vi "Register Task.vi"(8 "error in (no error)":errorcluster, 9 "Task ID":string, 10 "EnQr":refnum<class "Message Enqueuer.lvclass">, 11 "VolatusCore in":refnum<class "VolatusCore.lvclass">) -> (0 "error out":errorcluster, 3 "VolatusCore out":refnum<class "VolatusCore.lvclass">)   [LabVIEW 2020, in "Volatus.lvlib" / "VolatusCore.lvclass"]
uses:
  VolatusCore.lvclass
  VolatusCore.lvclass/VolatusCore.ctl
  <vilib>/Utility/miscctls.llb/LVMapReplaceAction.ctl
  <vilib>/ActorFramework/Message Enqueuer/Message Enqueuer.lvclass
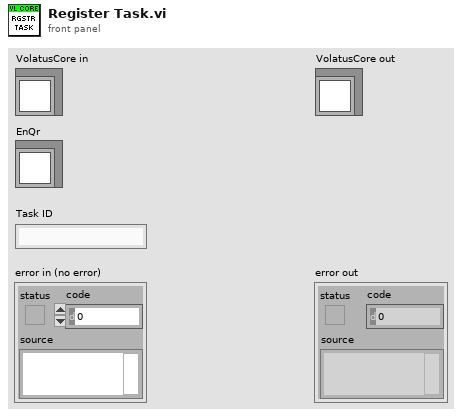
[diagram p1: front panel]
types:
  T1 = typedef "LVMapReplaceAction.ctl" = enum32{"Modify Entry only if found", "Add or Modify Entry", "Delete Entry"}
  T2 = map{string, refnum<class "Message Enqueuer.lvclass">}
  T3 = map{refnum<class "Message Enqueuer.lvclass">, string}
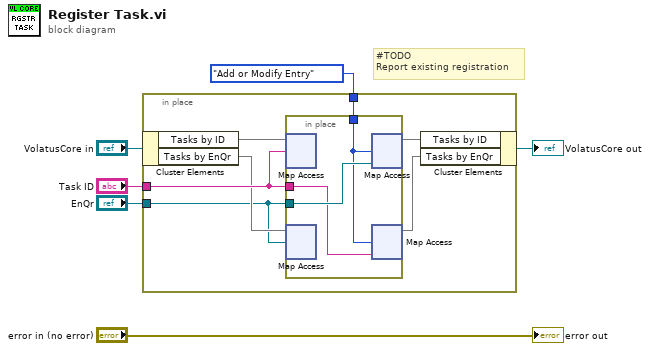
[diagram p0: block diagram]
diagram:
  # "#TODO\nReport existing registration"
  n1 = in-place {
    in-place-border: "Task ID" -> [w12]
    in-place-border: "EnQr" -> [w10]
    in-place-border: LVMapReplaceAction."Add or Modify Entry" ("action") -> [w9]
    n2 = in-place-cluster #1("VolatusCore in") -> ("Tasks by ID"=w13:T2, "Tasks by EnQr"=w11:T3)
    n3 = in-place {
      in-place-border: w12 -> [w15]
      in-place-border: w10 -> [w16]
      in-place-border: w9 -> [w14]
      n4 = in-place-map #2(w13, w12) -> ()  [unwired: 1 in, 2 out]
      n5 = in-place-map #3(w11, w10) -> ()  [unwired: 1 in, 2 out]
      n6 = in-place-map #2(w16, w14) -> (w8:T2)  [unwired: 2 out]
      n7 = in-place-map #3(w15, w14) -> (w7:T3)  [unwired: 2 out]
    }
    n8 = in-place-cluster #1("Tasks by ID"=w8, "Tasks by EnQr"=w7) -> (→"VolatusCore out":refnum<class "VolatusCore.lvclass">)
  }
  "error out" <- "error in (no error)"
